vi "CSUMetClient.vi"() -> (0 "Time Of Value (s)":dbl format="%#.1f", 1 "Error":bool, 2 "RawPressure/mBar":dbl)   [LabVIEW 2016]
panel:
  out "ComputerTime":timestamp
  out "MetTimeStamp":timestamp
  out "data out":string
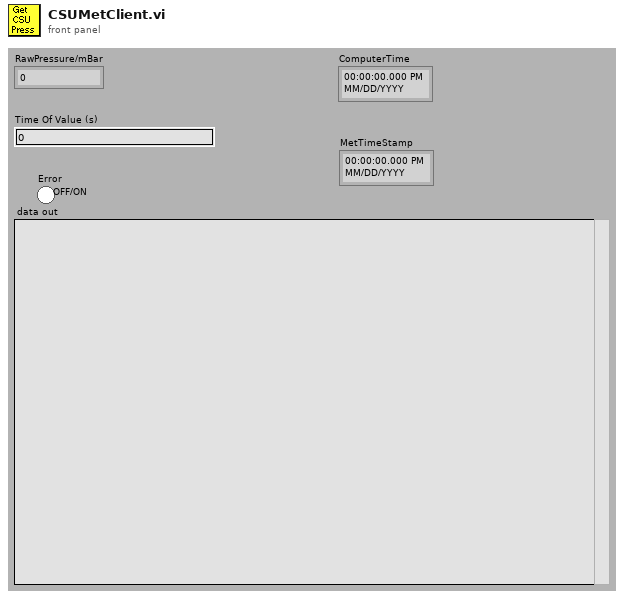
[diagram p1: front panel]
types:
  T1 = cluster{"second":i32, "minute":i32, "hour":i32, "day of month":i32, "month":i32, "year":i32, "day of week":i32, "day of year":i32, "is DST":i32}
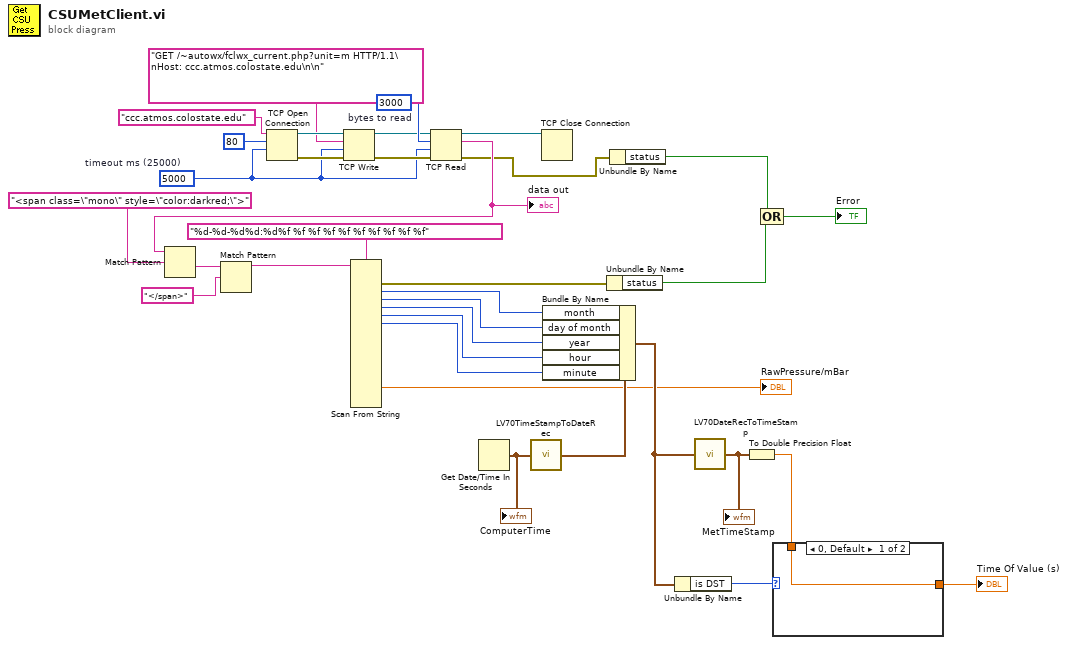
[diagram p0: block diagram]
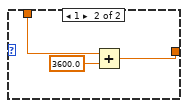
[diagram p2: hidden frame]
diagram:
  w2 = 5000  # timeout ms (25000)
  w27 = 3000  # bytes to read
  n1 = TCP Open Connection(address="ccc.atmos.colostate.edu", remote port or service name=u16 80 ("remote port"), timeout ms (60000)=w2) -> (connection ID=w32:refnum<k5>, error out=w30:errorcluster)  [unwired: 1 in, 1 out]
  n2 = TCP Write(connection ID=w32, data in="GET /~autowx/fclwx_current.php?unit=m HTTP/1.1\nHost: ccc.atmos.colostate.edu\n\n", error in (no error)=w30, 9:w2) -> (connection ID out=w26:refnum<k5>, error out=w29:errorcluster)  [unwired: 1 out]
  n3 = TCP Read(connection ID=w26, bytes to read=w27, error in (no error)=w29, 9:w2) -> (connection ID out=w28:refnum<k5>, data out=w13:string, error out=w1:errorcluster)  [unwired: 1 out]
  "data out" <- w13
  n4 = Match Pattern(string=w13, regular expression="<span class=\"mono\" style=\"color:darkred;\">") -> (after substring=w15:string)  [unwired: 4 out]
  n5 = Match Pattern(string=w15, regular expression="</span>") -> (before substring=w12:string)  [unwired: 4 out]
  n6 = Scan From String(format string="%d-%d-%d%d:%d%f %f %f %f %f %f %f %f %f %f", input string=w12) -> (error out=w9:errorcluster, output 1=w4:i32, output 2=w5:i32, output 3=w6:i32, output 4=w7:i32, output 5=w8:i32, output 13=→"RawPressure/mBar":dbl)  [unwired: 2 in, 26 out]
  n7 = Get Date/Time In Seconds() -> (seconds since 1Jan1904=w17:timestamp)
  "ComputerTime" <- w17
  n8 = call <vilib>:"LV70TimeStampToDateRec.vi"("time stamp"=w17) -> ("date time rec"=w25:T1)
  n9 = TCP Close Connection(connection ID=w28) -> ()  [unwired: 1 in, 3 out]
  n10 = Bundle By Name(cluster=w25, "month"=w4, "day of month"=w5, "year"=w6, "hour"=w7, "minute"=w8) -> (w23:T1)
  n11 = Unbundle By Name(w9) -> ("status"=w10:bool)
  n12 = Unbundle By Name(w1) -> ("status"=w20:bool)
  n13 = Unbundle By Name(w23) -> ("is DST"=w22:i32)
  n14 = call <vilib>:"LV70DateRecToTimeStamp.vi"("date time rec"=w23) -> ("Time Stamp"=w24:timestamp)
  "MetTimeStamp" <- w24
  n15 = To Double Precision Float(number=w24) -> (double precision float=w21:dbl)
  n16 = Compound Arithmetic op=OR(w20, w10) -> (→"Error":bool)
  n17 = case shown="0, Default" w22 {
    tunnel: w21 -> [w35 w38]
    tunnel: [w35 w36] -> w18
    frame 0, Default {
    }
    frame 1 {
      n18 = Add(x=w38, y=3600.0) -> (x+y=w36:dbl)
    }
  }
  "Time Of Value (s)" <- w18
